vi "SUB measure_Peak2Noise.vi"(1 "Cluster":cluster{"width":i32, "fc":dbl}={"width"=3, "fc"=459.016393442623}, 2 "Noise":waveform(dbl), 3 "Signal":waveform(dbl)) -> (0 "S/R":dbl)   [LabVIEW 2017]
panel:
  out "Array":dbl[](array[numeric])
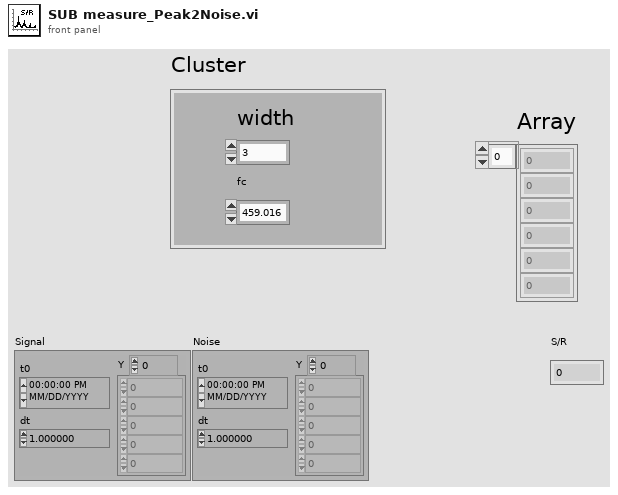
[diagram p1: front panel]
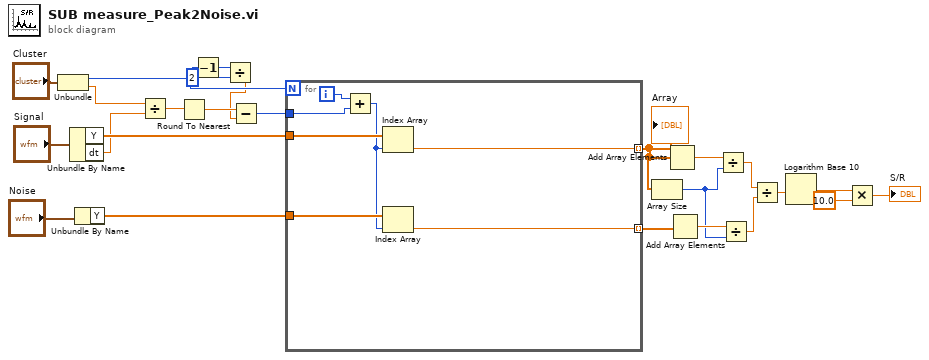
[diagram p0: block diagram]
diagram:
  n1 = Unbundle("Cluster") -> ("width"=w4:i32, "fc"=w7:dbl)
  n2 = Unbundle By Name("Signal") -> ("Y"=w22:dbl[], "dt"=w10:dbl)
  n3 = Unbundle By Name("Noise") -> ("Y"=w21:dbl[])
  n4 = Divide(x=w7, y=w10) -> (x/y=w23:dbl)
  n5 = Round To Nearest(number=w23) -> (nearest integer value=w20:dbl)
  n6 = Decrement(x=w4) -> (x-1=w3:i32)
  n7 = Divide(x=w3, y=2) -> (x/y=w1:dbl)
  n8 = Subtract(x=w20, y=w1) -> (x-y=w9:i64)
  n9 = for {
    N: w4 -> [_]
    tunnel: w22 -> [w32]
    tunnel: w21 -> [w31]
    tunnel: w9 -> [w29]
    tunnel: [w27] -> w6 mode=indexing
    tunnel: [w26] -> w14 mode=indexing
    i -> [w30]
    n10 = Add(x=w30, y=w29) -> (x+y=w28:i64)
    n11 = Index Array(array=w32, index=w28) -> (element=w27:dbl)
    n12 = Index Array(array=w31, index=w28) -> (element=w26:dbl)
  }
  "Array" <- w6
  n13 = Array Size(array=w6) -> (size(s)=w5:i32)
  n14 = Add Array Elements(numeric array=w6) -> (sum=w19:dbl)
  n15 = Add Array Elements(numeric array=w14) -> (sum=w15:dbl)
  n16 = Divide(x=w19, y=w5) -> (x/y=w12:dbl)
  n17 = Divide(x=w15, y=w5) -> (x/y=w13:dbl)
  n18 = Divide(x=w12, y=w13) -> (x/y=w11:dbl)
  n19 = Logarithm Base 10(1:w11) -> (0:w18:dbl)
  n20 = Multiply(x=w18, y=10.0) -> (x*y=→"S/R":dbl)
